vi "KrakenConfigPID.vi"(6 "PID Slot":i32, 7 "Error (in)":errorcluster, 8 "DeviceConfiguration":T1={"Future Proof Configs"=FALSE, "MotorOutputInverted"=0, "MotorOutputNeutralMode"=0, "MotorOutputDutyCycleNeutralDeadband"=0.0, "MotorOutputPeakForwardDutyCycle"=1.0, "MotorOutputPeakReverseDutyCycle"=-1.0, "CurrentLimitsStatorCurrentLimit"=0.0, "CurrentLimitsStatorCurrentLimitEnable"=FALSE, "CurrentLimitsSupplyCurrentLimit"=0.0, "CurrentLimitsSupplyCurrentLimitEnable"=FALSE, "CurrentLimitsSupplyCurrentThreshold"=0.0, "CurrentLimitsSupplyTimeThreshold"=0.0, "VoltageSupplyVoltageTimeConstant"=0.0, "VoltagePeakForwardVoltage"=16.0, "VoltagePeakReverseVoltage"=-16.0, "TorqueCurrentPeakForwardTorqueCurrent"=800.0, "TorqueCurrentPeakReverseTorqueCurrent"=-800.0, "TorqueCurrentTorqueNeutralDeadband"=0.0, "FeedbackFeedbackRotorOffset"=0.0, "FeedbackSensorToMechanismRatio"=1.0, "FeedbackRotorToSensorRatio"=1.0, "FeedbackFeedbackSensorSource"=0, "FeedbackFeedbackRemoteSensorID"=0, "DifferentialSensorsDifferentialSensorSource"=0, "DifferentialSensorsDifferentialTalonFXSensorID"=0, "DifferentialSensorsDifferentialRemoteSensorID"=0, "DifferentialConstantsPeakDifferentialDutyCycle"=2.0, "DifferentialConstantsPeakDifferentialVoltage"=32.0, "DifferentialConstantsPeakDifferentialTorqueCurrent"=1600.0, "OpenLoopRampsDutyCycleOpenLoopRampPeriod"=0.0, "OpenLoopRampsVoltageOpenLoopRampPeriod"=0.0, "OpenLoopRampsTorqueOpenLoopRampPeriod"=0.0, "ClosedLoopRampsDutyCycleClosedLoopRampPeriod"=0.0, "ClosedLoopRampsVoltageClosedLoopRampPeriod"=0.0, "ClosedLoopRampsTorqueClosedLoopRampPeriod"=0.0, "HardwareLimitSwitchForwardLimitType"=0, "HardwareLimitSwitchForwardLimitAutosetPositionEnable"=FALSE, "HardwareLimitSwitchForwardLimitAutosetPositionValue"=0.0, "HardwareLimitSwitchForwardLimitEnable"=TRUE, "HardwareLimitSwitchForwardLimitSource"=0, "HardwareLimitSwitchForwardLimitRemoteSensorID"=0, "HardwareLimitSwitchReverseLimitType"=0, "HardwareLimitSwitchReverseLimitAutosetPositionEnable"=FALSE, "HardwareLimitSwitchReverseLimitAutosetPositionValue"=0.0, "HardwareLimitSwitchReverseLimitEnable"=TRUE, "HardwareLimitSwitchReverseLimitSource"=0, "HardwareLimitSwitchReverseLimitRemoteSensorID"=0, "AudioBeepOnBoot"=TRUE, "AudioBeepOnConfig"=TRUE, "AudioAllowMusicDurDisable"=FALSE, "SoftwareLimitSwitchForwardSoftLimitEnable"=FALSE, "SoftwareLimitSwitchReverseSoftLimitEnable"=FALSE, "SoftwareLimitSwitchForwardSoftLimitThreshold"=0.0, "SoftwareLimitSwitchReverseSoftLimitThreshold"=0.0, "MotionMagicMotionMagicCruiseVelocity"=0.0, "MotionMagicMotionMagicAcceleration"=0.0, "MotionMagicMotionMagicJerk"=0.0, "MotionMagicMotionMagicExpo_kV"=0.0, "MotionMagicMotionMagicExpo_kA"=0.0, "CustomParamsCustomParam0"=0, "CustomParamsCustomParam1"=0, "ClosedLoopGeneralContinuousWrap"=FALSE, "Slot0kP"=0.0, "Slot0kI"=0.0, "Slot0kD"=0.0, "Slot0kS"=0.0, "Slot0kV"=0.0, "Slot0kA"=0.0, "Slot0kG"=0.0, "Slot0GravityType"=0, "Slot0StaticFeedforwardSign"=0, "Slot1kP"=0.0, "Slot1kI"=0.0, "Slot1kD"=0.0, "Slot1kS"=0.0, "Slot1kV"=0.0, "Slot1kA"=0.0, "Slot1kG"=0.0, "Slot1GravityType"=0, "Slot1StaticFeedforwardSign"=0, "Slot2kP"=0.0, "Slot2kI"=0.0, "Slot2kD"=0.0, "Slot2kS"=0.0, "Slot2kV"=0.0, "Slot2kA"=0.0, "Slot2kG"=0.0, "Slot2GravityType"=0, "Slot2StaticFeedforwardSign"=0} {"MotorOutputInverted" items=["CounterClockwise_Positive", "Clockwise_Positive"]; "MotorOutputNeutralMode" items=["Coast", "Brake"]; "FeedbackFeedbackSensorSource" items=["RotorSensor", "RemoteCANcoder", "RemotePigeon2_Yaw", "RemotePigeon2_Pitch", "RemotePigeon2_Roll", "FusedCANcoder", "SyncCANcoder"]; "DifferentialSensorsDifferentialSensorSource" items=["Disabled", "RemoteTalonFX_Diff", "RemotePigeon2_Yaw", "RemotePigeon2_Pitch", "RemotePigeon2_Roll", "RemoteCANcoder"]; "HardwareLimitSwitchForwardLimitType" items=["NormallyOpen", "NormallyClosed"]; "HardwareLimitSwitchForwardLimitSource" items=["LimitSwitchPin"=0, "RemoteTalonFX"=1, "RemoteCANifier"=2, "RemoteCANcoder"=4, "Disabled"=3]; "HardwareLimitSwitchReverseLimitType" items=["NormallyOpen", "NormallyClosed"]; "HardwareLimitSwitchReverseLimitSource" items=["LimitSwitchPin"=0, "RemoteTalonFX"=1, "RemoteCANifier"=2, "RemoteCANcoder"=4, "Disabled"=3]; "Slot0GravityType" items=["Elevator_Static", "Arm_Cosine"]; "Slot0StaticFeedforwardSign" items=["UseVelocitySign", "UseClosedLoopSign"]; "Slot1GravityType" items=["Elevator_Static", "Arm_Cosine"]; "Slot1StaticFeedforwardSign" items=["UseVelocitySign", "UseClosedLoopSign"]; "Slot2GravityType" items=["Elevator_Static", "Arm_Cosine"]; "Slot2StaticFeedforwardSign" items=["UseVelocitySign", "UseClosedLoopSign"]}, 9 "PID Parameters":cluster{"Kp":dbl, "Ki":dbl, "Kd":dbl}, 10 "DeviceReference (in)":T2) -> (0 "Error (out)":errorcluster, 2 "DeviceConfiguration(OUT)":T1, 3 "DeviceReference (out)":T2)   [LabVIEW 2023]
doc: "Wrapper for configuring the PID on a Talon FX motor controller."
uses:
  <vilib>/Rock Robotics/WPI/ThirdParty/Phoenix6/DeviceReference.ctl
  5ec5a0a5-e256-4685-9647-f7ac00e8f22e.vi
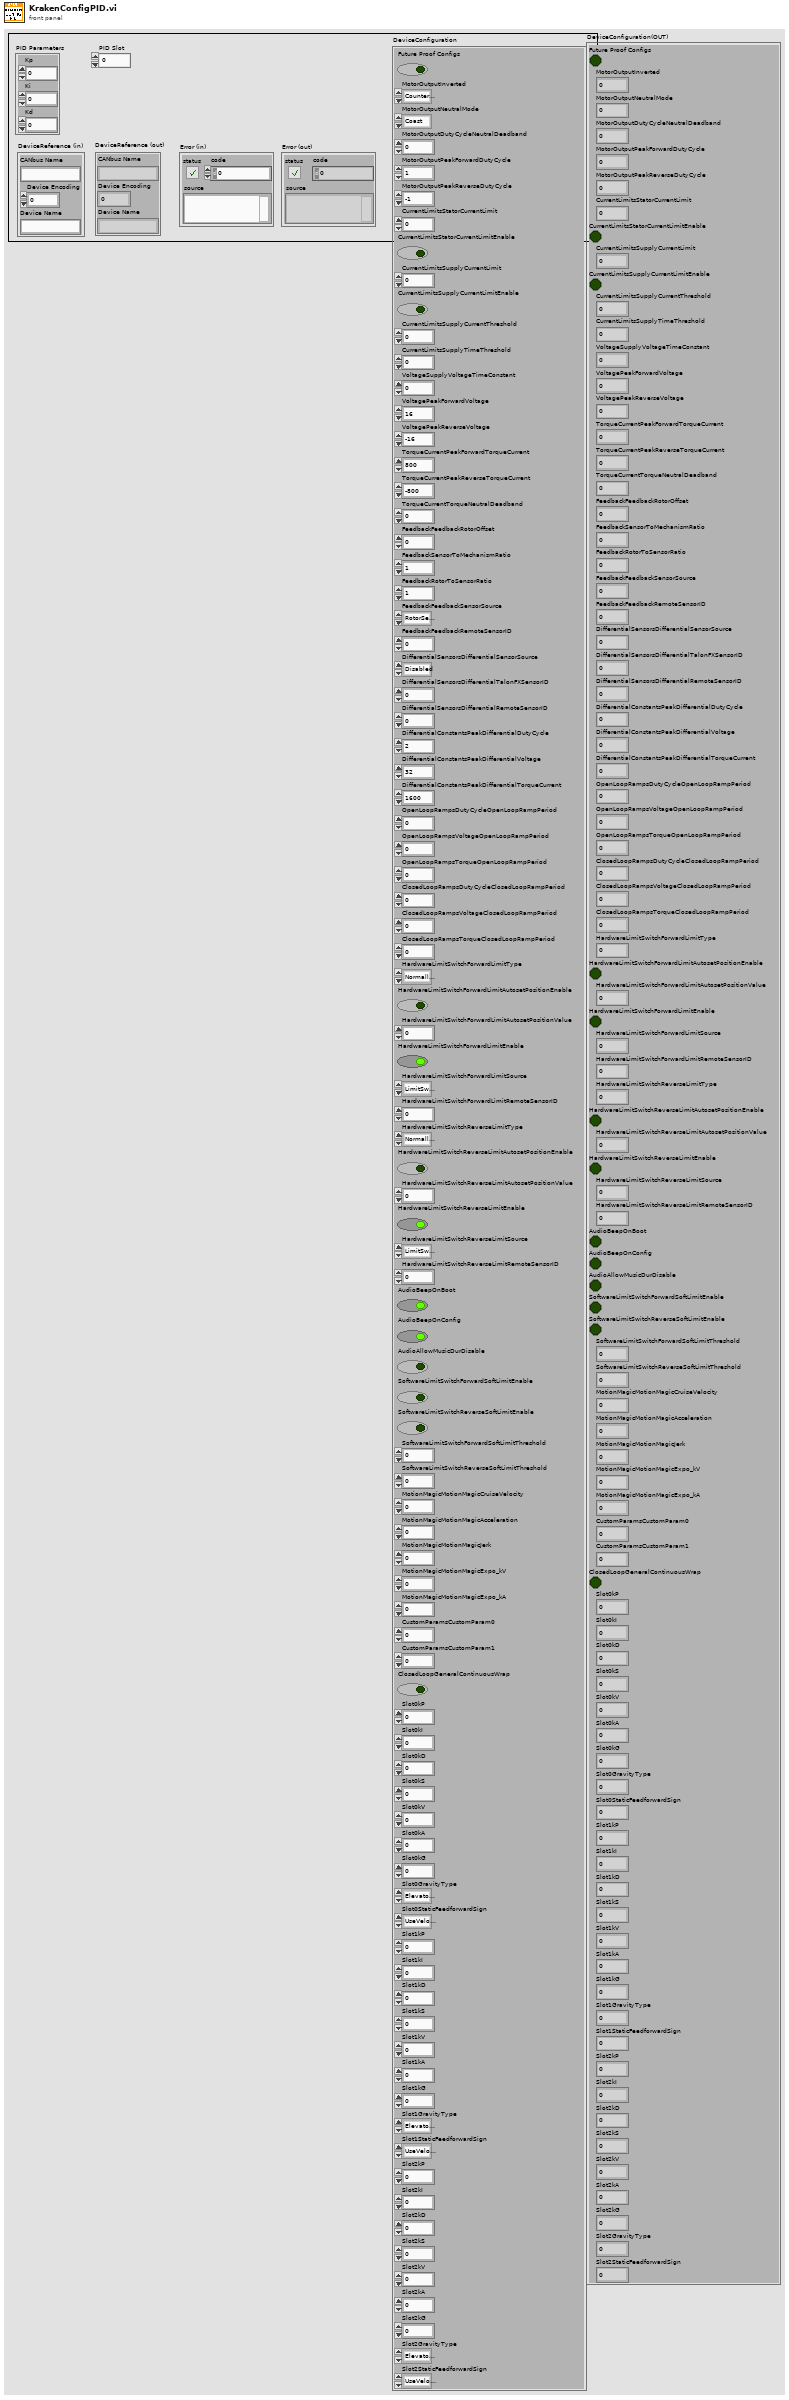
[diagram p1: front panel]
types:
  T1 = cluster{"Future Proof Configs":bool, "MotorOutputInverted":u16, "MotorOutputNeutralMode":u16, "MotorOutputDutyCycleNeutralDeadband":dbl, "MotorOutputPeakForwardDutyCycle":dbl, "MotorOutputPeakReverseDutyCycle":dbl, "CurrentLimitsStatorCurrentLimit":dbl, "CurrentLimitsStatorCurrentLimitEnable":bool, "CurrentLimitsSupplyCurrentLimit":dbl, "CurrentLimitsSupplyCurrentLimitEnable":bool, "CurrentLimitsSupplyCurrentThreshold":dbl, "CurrentLimitsSupplyTimeThreshold":dbl, "VoltageSupplyVoltageTimeConstant":dbl, "VoltagePeakForwardVoltage":dbl, "VoltagePeakReverseVoltage":dbl, "TorqueCurrentPeakForwardTorqueCurrent":dbl, "TorqueCurrentPeakReverseTorqueCurrent":dbl, "TorqueCurrentTorqueNeutralDeadband":dbl, "FeedbackFeedbackRotorOffset":dbl, "FeedbackSensorToMechanismRatio":dbl, "FeedbackRotorToSensorRatio":dbl, "FeedbackFeedbackSensorSource":u16, "FeedbackFeedbackRemoteSensorID":i16, "DifferentialSensorsDifferentialSensorSource":u16, "DifferentialSensorsDifferentialTalonFXSensorID":i16, "DifferentialSensorsDifferentialRemoteSensorID":i16, "DifferentialConstantsPeakDifferentialDutyCycle":dbl, "DifferentialConstantsPeakDifferentialVoltage":dbl, "DifferentialConstantsPeakDifferentialTorqueCurrent":dbl, "OpenLoopRampsDutyCycleOpenLoopRampPeriod":dbl, "OpenLoopRampsVoltageOpenLoopRampPeriod":dbl, "OpenLoopRampsTorqueOpenLoopRampPeriod":dbl, "ClosedLoopRampsDutyCycleClosedLoopRampPeriod":dbl, "ClosedLoopRampsVoltageClosedLoopRampPeriod":dbl, "ClosedLoopRampsTorqueClosedLoopRampPeriod":dbl, "HardwareLimitSwitchForwardLimitType":u16, "HardwareLimitSwitchForwardLimitAutosetPositionEnable":bool, "HardwareLimitSwitchForwardLimitAutosetPositionValue":dbl, "HardwareLimitSwitchForwardLimitEnable":bool, "HardwareLimitSwitchForwardLimitSource":u16, "HardwareLimitSwitchForwardLimitRemoteSensorID":i16, "HardwareLimitSwitchReverseLimitType":u16, "HardwareLimitSwitchReverseLimitAutosetPositionEnable":bool, "HardwareLimitSwitchReverseLimitAutosetPositionValue":dbl, "HardwareLimitSwitchReverseLimitEnable":bool, "HardwareLimitSwitchReverseLimitSource":u16, "HardwareLimitSwitchReverseLimitRemoteSensorID":i16, "AudioBeepOnBoot":bool, "AudioBeepOnConfig":bool, "AudioAllowMusicDurDisable":bool, "SoftwareLimitSwitchForwardSoftLimitEnable":bool, "SoftwareLimitSwitchReverseSoftLimitEnable":bool, "SoftwareLimitSwitchForwardSoftLimitThreshold":dbl, "SoftwareLimitSwitchReverseSoftLimitThreshold":dbl, "MotionMagicMotionMagicCruiseVelocity":dbl, "MotionMagicMotionMagicAcceleration":dbl, "MotionMagicMotionMagicJerk":dbl, "MotionMagicMotionMagicExpo_kV":dbl, "MotionMagicMotionMagicExpo_kA":dbl, "CustomParamsCustomParam0":i16, "CustomParamsCustomParam1":i16, "ClosedLoopGeneralContinuousWrap":bool, "Slot0kP":dbl, "Slot0kI":dbl, "Slot0kD":dbl, "Slot0kS":dbl, "Slot0kV":dbl, "Slot0kA":dbl, "Slot0kG":dbl, "Slot0GravityType":u16, "Slot0StaticFeedforwardSign":u16, "Slot1kP":dbl, "Slot1kI":dbl, "Slot1kD":dbl, "Slot1kS":dbl, "Slot1kV":dbl, "Slot1kA":dbl, "Slot1kG":dbl, "Slot1GravityType":u16, "Slot1StaticFeedforwardSign":u16, "Slot2kP":dbl, "Slot2kI":dbl, "Slot2kD":dbl, "Slot2kS":dbl, "Slot2kV":dbl, "Slot2kA":dbl, "Slot2kG":dbl, "Slot2GravityType":u16, "Slot2StaticFeedforwardSign":u16}
  T2 = typedef "DeviceReference.ctl" = cluster{"CANbus Name":string, "Device Encoding":u32, "Device Name":string}
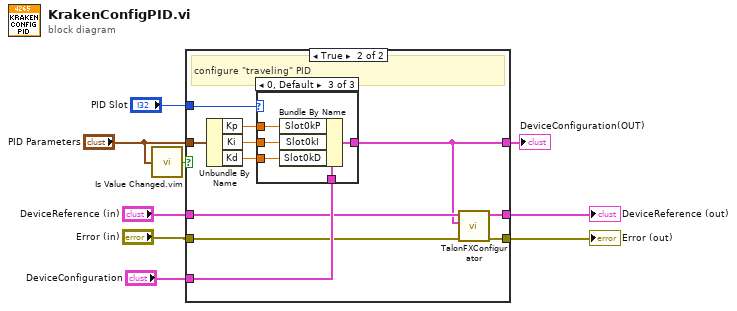
[diagram p0: block diagram]
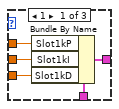
[diagram p3: hidden frame]
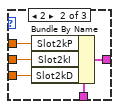
[diagram p4: hidden frame]
diagram:
  n1 = call "Is Value Changed.vim"("value"="PID Parameters") -> ("changed or first call?"=w5:bool)
  n2 = case shown="True" w5 {
    tunnel: "PID Parameters" -> [_ w22]
    tunnel: "DeviceReference (in)" -> [w12 w14]
    tunnel: "Error (in)" -> [w11 w15]
    tunnel: [w12 w14] -> w7
    tunnel: [w11 w16] -> w8
    tunnel: "PID Slot" -> [_ w17]
    tunnel: "DeviceConfiguration" -> [w10 w21]
    tunnel: [w10 w13] -> w1
    frame False {
    }
    frame True {
      # "configure \"traveling\" PID"
      n3 = Unbundle By Name(w22) -> ("Kp"=w20:dbl, "Ki"=w19:dbl, "Kd"=w18:dbl)
      n4 = case shown="0, Default" w17 {
        tunnel: w21 -> [w27 w32 w37]
        tunnel: w20 -> [w24 w31 w36]
        tunnel: w19 -> [w25 w30 w35]
        tunnel: w18 -> [w26 w29 w34]
        tunnel: [w23 w28 w33] -> w13
        frame 1 {
          n5 = Bundle By Name(cluster=w27, "Slot1kP"=w24, "Slot1kI"=w25, "Slot1kD"=w26) -> (w23:T1)
        }
        frame 2 {
          n6 = Bundle By Name(cluster=w32, "Slot2kP"=w31, "Slot2kI"=w30, "Slot2kD"=w29) -> (w28:T1)
        }
        frame 0, Default {
          n7 = Bundle By Name(cluster=w37, "Slot0kP"=w36, "Slot0kI"=w35, "Slot0kD"=w34) -> (w33:T1)
        }
      }
      n8 = call <vilib>:"TalonFXConfigurator.vi"("error in"=w15, "DeviceConfiguration"=w13, "DeviceReference"=w14) -> ("error out"=w16:errorcluster)  [unwired: 8 in]
    }
  }
  "Error (out)" <- w8
  "DeviceReference (out)" <- w7
  "DeviceConfiguration(OUT)" <- w1
